vi "Insert Set Item Property.vi"(7 "Constants VI":path, 8 "error in (no error)":errorcluster, 9 "Property Info":T1, 10 "Wires[]":refnum<vi>[](array[refnum]), 11 "VI Refnum":refnum<vi>) -> (0 "error out":errorcluster, 3 "VI Refnum out":refnum<vi>)   [LabVIEW 2017, in "NIVS_Consolidated_CDW_MetaDataObj.lvclass"]
doc: "Inserts the NI VeriStand - Set Item Property VI on the selected wires and creates the value and the property name from the Constants.vi global."
uses:
  NIVS_Consolidated_CDW_MetaDataObj.lvclass
  Property Information.ctl
  <vilib>/Utility/QuickDropSupport/QuickDrop Plugin Data ver1.ctl
  <vilib>/Utility/traverseref.llb/TRef TravTarget.ctl
  <vilib>/Utility/traverseref.llb/VI Scripting - Traverse.lvlib
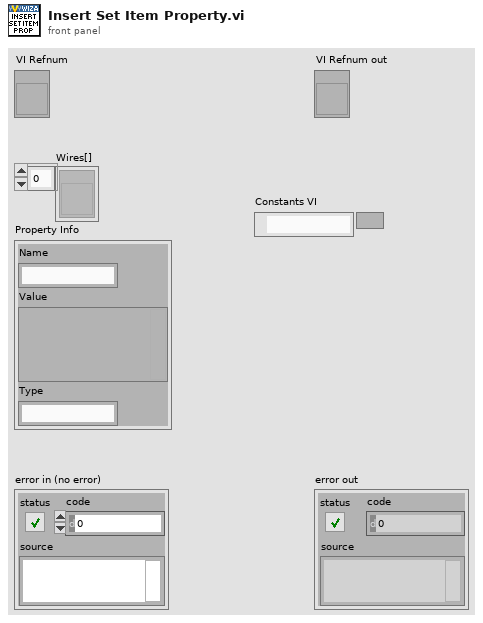
[diagram p1: front panel]
types:
  T1 = typedef "NIVS_Consolidated_CDW_MetaDataObj.lvclass/Property Information.ctl" = cluster{"Name":string, "Value":variant, "Type":string}
  T2 = typedef "TRef TravTarget.ctl" = enum16{"FP", "BD", "Other"}
  T3 = typedef "QuickDrop Plugin Data ver1.ctl" = cluster{"FP.IsFrontMost?":bool, "Project VI Path":path, "Palette Object Name":string}
  T4 = cluster{"VIPath":path, "Menu Name":string, "Selector Name":string}[]
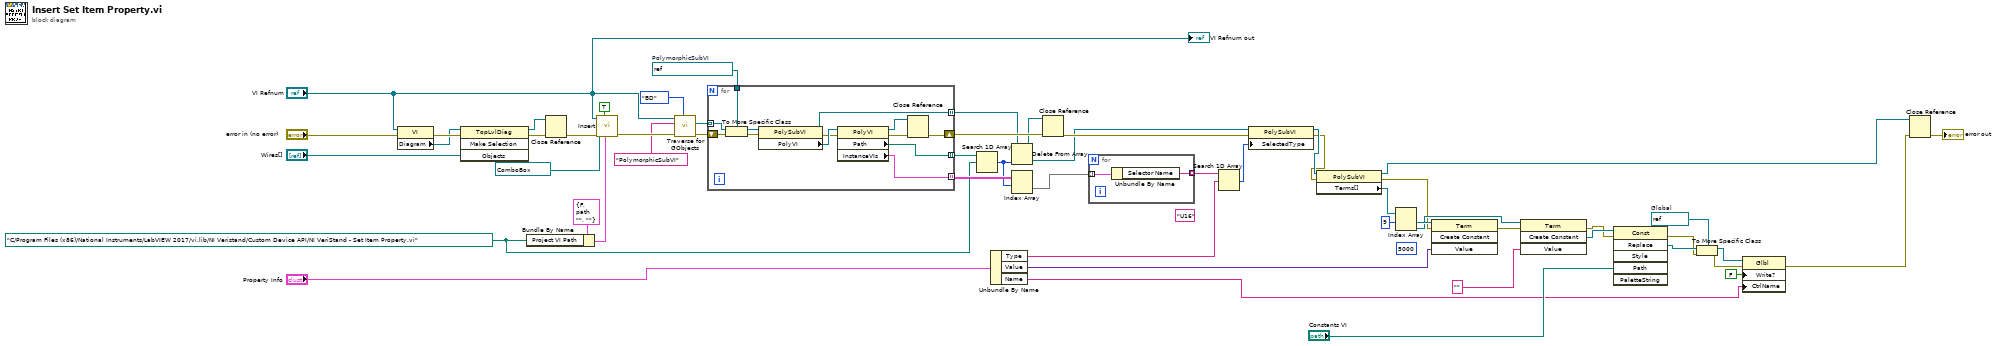
[diagram p0: block diagram]
diagram:
  w16 = refnum<vi> refnum  # Global
  (unwired) u16 5000
  w28 = path "C:/Program Files (x86)/National Instruments/LabVIEW 2017/vi.lib/NI Veristand/Custom Device API/NI VeriStand - Set Item Property.vi" ("path")
  w36 = refnum<vi> refnum  # PolymorphicSubVI
  (unwired) "U16"
  n1 = property class="VI"(reference="VI Refnum", error in="error in (no error)") -> (error out=w54:errorcluster, "Diagram"=w53:refnum<vi>)  [unwired: 1 out]
  n2 = invoke class="TopLvlDiag" method="Make Selection"(reference=w53, error in=w54, "Objects"="Wires[]") -> (reference out=w51:refnum<vi>, error out=w52:errorcluster)  [unwired: 1 in, 2 out]
  n3 = Bundle By Name(cluster=T3 {"FP.IsFrontMost?"=FALSE, "Project VI Path"=path "", "Palette Object Name"=""} ("Quick Drop Plugin Data"), "Project VI Path"=w28) -> (w47:T3)
  n4 = Close Reference(reference=w51, error in (no error)=w52) -> (error out=w30:errorcluster)
  n5 = call <resource>:"Insert.vi"("Variant in"=w47, "Shift Pressed?"=TRUE, "error in (no error)"=w30, "QD Combo Box Ref"=refnum<vi> refnum, "QD Launch VI Ref"="VI Refnum") -> ("error out"=w46:errorcluster)  [unwired: 5 in, 1 out]
  n6 = call <vilib>:"Traverse for GObjects.vi"("Traverse Target"=TRef_TravTarget."BD", "error in (no error)"=w46, "Class Name"="PolymorphicSubVI", "VI Refnum"="VI Refnum") -> ("error out"=w43:errorcluster, "References"=w37:refnum<vi>[])  [unwired: 4 in, 2 out]
  n7 = for {
    tunnel: w37 -> [w68] mode=indexing
    tunnel: w36 -> [w67]
    shift-right: [w57] -> w41
    shift-left: w43 -> [w65]
    tunnel: [w61] -> w42 mode=indexing
    tunnel: [w63] -> w35 mode=indexing
    tunnel: [w58] -> w34 mode=indexing
    n8 = To More Specific Class(target class=w67, reference=w68, error in=w65) -> (specific class reference=w66:refnum<vi>, error out=w64:errorcluster)
    n9 = property class="PolySubVI"(reference=w66, error in=w64) -> (reference out=w63:refnum<vi>, error out=w60:errorcluster, "PolyVI"=w62:refnum<vi>)
    n10 = property class="PolyVI"(reference=w62, error in=w60) -> (reference out=w56:refnum<vi>, error out=w59:errorcluster, "Path"=w61:path, "InstanceVIs"=w58:T4)
    n11 = Close Reference(reference=w56, error in (no error)=w59) -> (error out=w57:errorcluster)
  }
  n12 = Search 1D Array(1D array=w42, element=w28) -> (index of element=w32:i32)  [unwired: 1 in]
  n13 = Unbundle By Name("Property Info") -> ("Type"=w8:string, "Value"=w7:variant, "Name"=w6:string)
  n14 = Delete From Array(array=w35, index=w32) -> (deleted portion=w38:refnum<vi>, array with subset deleted=w40:refnum<vi>[])  [unwired: 1 in]
  n15 = Index Array(array=w34, index (row)=w32) -> (element=w33:T4)  [unwired: 1 in]
  n16 = Close Reference(reference=w40, error in (no error)=w41) -> (error out=w39:errorcluster)
  n17 = for {
    tunnel: w33 -> [w70] mode=indexing
    tunnel: [w69] -> w50 mode=indexing
    n18 = Unbundle By Name(w70) -> ("Selector Name"=w69:string)
  }
  n19 = Search 1D Array(1D array=w50, element=w8) -> (index of element=w49:i32)  [unwired: 1 in]
  n20 = property class="PolySubVI"(reference=w38, error in=w39, "SelectedType"=w49) -> (reference out=w13:refnum<vi>, error out=w11:errorcluster)
  n21 = property class="PolySubVI"(reference=w13, error in=w11) -> (reference out=w12:refnum<vi>, error out=w5:errorcluster, "Terms[]"=w24:refnum<vi>[])
  n22 = Index Array(array=w24, index #1=9 ("index")) -> (element #1=w22:refnum<vi>, element #2=w19:refnum<vi>)  [unwired: 1 in]
  n23 = invoke class="Term" method="Create Constant"(reference=w22, error in=w5, "Value"=w7) -> (error out=w20:errorcluster)  [unwired: 1 in, 3 out]
  n24 = invoke class="Term" method="Create Constant"(reference=w19, error in=w20, "Value"="") -> (error out=w4:errorcluster, "Create Constant"=w18:refnum<vi>)  [unwired: 1 in, 2 out]
  n25 = invoke class="Const" method="Replace"(reference=w18, error in=w4, "Path"="Constants VI") -> (error out=w3:errorcluster, "Replace"=w17:refnum<vi>)  [unwired: 3 in, 4 out]
  n26 = To More Specific Class(target class=w16, reference=w17, error in=w3) -> (specific class reference=w15:refnum<vi>, error out=w2:errorcluster)
  n27 = property class="Glbl"(reference=w15, error in=w2, "Write?"=FALSE, "CtrlName"=w6) -> (error out=w1:errorcluster)  [unwired: 1 out]
  n28 = Close Reference(reference=w12, error in (no error)=w1) -> (error out=→"error out":errorcluster)
  "VI Refnum out" <- "VI Refnum"
